vi "tablePartsTracking.vi"(8 "error in (no error)":errorcluster, 10 "Table in":refnum<vi>, 11 "reference in":refnum<class "Project Panels.lvclass">) -> (0 "error out":errorcluster, 3 "reference out":refnum<class "Project Panels.lvclass">)   [LabVIEW 2015, in "Project Panels.lvclass"]
uses:
  Project Panels.lvclass
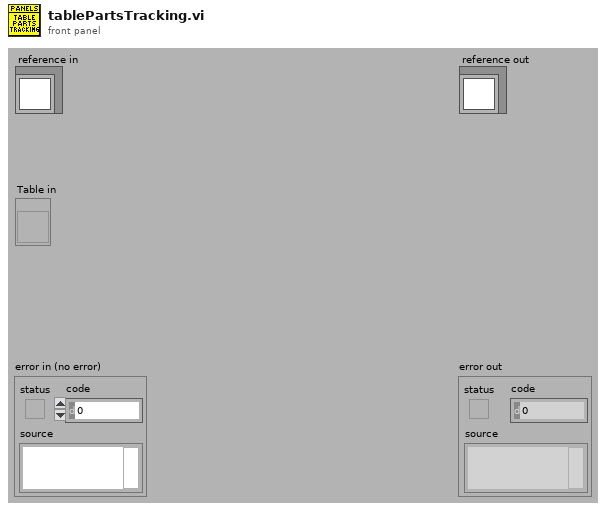
[diagram p1: front panel]
types:
  T1 = enum16{"User-specified Font", "Application Font", "System Font", "Dialog Font"}
  T2 = cluster{"Font Name:":string, "Size":i16, "Strikeout?":bool, "Italic?":bool, "Underline?":bool, "Outline?":bool, "Shadow?":bool, "Bold?":bool}
  T3 = typedef "Project Panels.lvclass/ObjectAttributesRef.ctl" = refnum<data-value>
  T4 = typedef "Project Panels.lvclass/ObjectAttributes.ctl" = cluster{"MyAttribute":dbl, "device_controller_ref":refnum<class "Devices Controller.lvclass">, "file_controller_ref":refnum<class "File Controller.lvclass">, "item_controller_ref":refnum<class "Items Controller.lvclass">, "item_tables":cluster{"checkIN":string[][], "checkOUT":string[][], "storage":string[][]}, "quickbook_table":cluster{"notes":string[][]}, "notification_controller_ref":refnum<class "Notification Controller.lvclass">, "partstracking_controller_ref":refnum<class "PartsTracking Controller.lvclass">, "product_tables":cluster{"k4b2":string[][], "fitmate":string[][], "RMR":string[][], "CPET":string[][], "BP":string[][], "PP":string[][], "k5":string[][], "bb-pft":string[][]}, "rowsColour":u32[], "low_resolution?":bool}
  T5 = cluster{"left":i16, "top":i16, "right":i16, "bottom":i16}
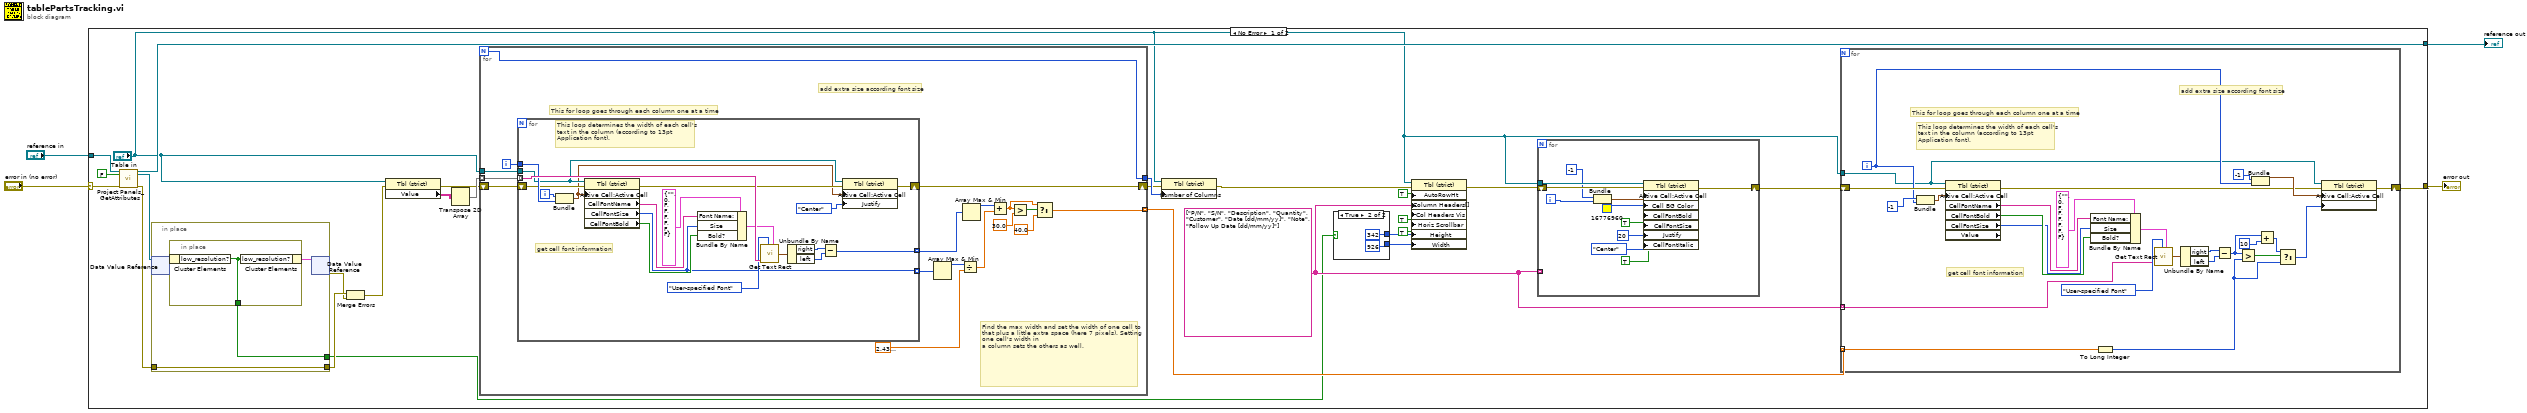
[diagram p0: block diagram]
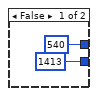
[diagram p2: hidden frame]
diagram:
  n1 = case shown="No Error" "error in (no error)" {
    selector: "error in (no error)" -> [w29 w115]
    tunnel: [w18 w115] -> w3
    tunnel: [w28 w114] -> w1
    tunnel: "reference in" -> [w31 w114]
    frame No Error {
      w14 = string[] ["P/N", "S/N", "Description", "Quantity", "Customer", "Date [dd/mm/yy]", "Note", "Follow Up Date [dd/mm/yy]"] ("Column Header Strings[]")
      n2 = call "Project Panels_GetAttributes.vi"("reference in"=w31, "return data? (T)"=FALSE, "error in (no error)"=w29) -> ("reference out"=w28:refnum<class "Project Panels.lvclass">, "attributes ref"=w6:T3, "error out"=w7:errorcluster)  [unwired: 13 in, 1 out]
      n3 = in-place {
        in-place-border: w7 -> [w33]
        in-place-border: [w33] -> w10
        in-place-border: [w32] -> w5
        n4 = in-place-dvr #1(w6) -> (w34:T4)  [unwired: 1 out]
        n5 = in-place {
          in-place-border: [w36] -> w32
          n6 = in-place-cluster #2(w34) -> ("low_resolution?"=w36:bool)
          n7 = in-place-cluster #2("low_resolution?"=w36) -> (w35:T4)
        }
        n8 = in-place-dvr #1(w35) -> (w9:errorcluster)  [unwired: 1 out]
      }
      n9 = Merge Errors(w10, w9) -> (w8:errorcluster)
      n10 = property on="Property Node" class="Tbl (strict)"(reference="Table in", error in=w8) -> (error out=w23:errorcluster, "Value"=w24:string[][])  [unwired: 1 out]
      n11 = Transpose 2D Array(2D array=w24) -> (transposed array=w25:string[][])
      n12 = for {
        N -> [w86]
        tunnel: w25 -> [w94] mode=indexing
        tunnel: [w86] -> w27
        tunnel: "Table in" -> [w85]
        shift-right: [w79] -> w26
        shift-left: w23 -> [w84]
        tunnel: [w78] -> w11 mode=indexing
        i -> [w92]
        # "add extra size according font size"
        # "Find the max width and set the width of one cell to that plus a little extra space (here 7 pixels). Setting one cell's width in\na column sets the others as well."
        # "This for loop goes through each column one at a time"
        n13 = for {
          tunnel: w94 -> [w113] mode=indexing
          tunnel: [w109] -> w93 mode=indexing
          tunnel: w92 -> [w104]
          tunnel: [w101] -> w90 mode=indexing
          tunnel: w85 -> [w96]
          shift-right: [w98] -> w79
          shift-left: w84 -> [w100]
          i -> [w103]
          # "get cell font information"
          # "This loop determines the width of each cell's\ntext in the column (according to 13pt\nApplication font)."
          n14 = Bundle(w103, w104) -> (w95:cluster{i32, i32})  [unwired: 1 in]
          n15 = property on="Property Node" class="Tbl (strict)"(reference=w96, error in=w100, "Active Cell:Active Cell"=w95) -> (error out=w99:errorcluster, "CellFontName"=w108:string, "CellFontSize"=w101:u32, "CellFontBold"=w107:bool)  [unwired: 1 out]
          n16 = Bundle By Name(cluster=T2 {"Font Name:"="", "Size"=0, "Strikeout?"=FALSE, "Italic?"=FALSE, "Underline?"=FALSE, "Outline?"=FALSE, "Shadow?"=FALSE, "Bold?"=FALSE} ("[user-specified font]"), "Font Name:"=w108, "Size"=w101, "Bold?"=w107) -> (w105:T2)
          n17 = call <vilib>:"Get Text Rect.vi"("desired font(Application)"=T1."User-specified Font", "text"=w113, "[user-specified font]"=w105) -> ("rect"=w112:T5)  [unwired: 6 in]
          n18 = Unbundle By Name(w112) -> ("right"=w111:i16, "left"=w110:i16)
          n19 = Subtract(x=w111, y=w110) -> (x-y=w109:i16)
          n20 = property on="Property Node" class="Tbl (strict)"(reference=w96, error in=w99, "Active Cell:Active Cell"=w95, "Justify"=enum16{"Left", "Center", "Right"}."Center" ("Active Cell:Cell Justification")) -> (error out=w98:errorcluster)  [unwired: 1 out]
        }
        n21 = Array Max & Min(array=w90) -> (max value=w89:u32)  [unwired: 3 out]
        n22 = Divide(x=w89, y=sgl 2.43) -> (x/y=w87:sgl)
        n23 = Array Max & Min(array=w93) -> (max value=w91:i16)  [unwired: 3 out]
        n24 = Add(x=w91, y=w87) -> (x+y=w80:sgl)
        n25 = Greater?(x=w80, y=sgl 30.0) -> (0:w82:bool)
        n26 = Select(t=w80, s=w82, f=sgl 40.0 ("y")) -> (s? t:f=w78:sgl)
      }
      n27 = property on="Property Node" class="Tbl (strict)"(reference="Table in", error in=w26, "Number of Columns"=w27) -> (error out=w19:errorcluster)  [unwired: 1 out]
      n28 = case shown="True" w5 {
        tunnel: [u32 540 ("Size:Height") u32 342 ("Size:Height")] -> w13
        tunnel: [u32 1413 ("Size:Width") u32 926 ("Size:Width")] -> w12
        frame False {
        }
        frame True {
        }
      }
      n29 = property on="Property Node" class="Tbl (strict)"(reference="Table in", error in=w19, "AutoRowHt"=TRUE ("Autosizing Row Height"), "Column Headers[]"=w14, "Col Headers Vis"=TRUE ("Visible Items:Column Headers Visible"), "Horiz Scrollbar"=TRUE ("Visible Items:Horizontal Scrollbar Visible"), "Height"=w13, "Width"=w12) -> (error out=w17:errorcluster)  [unwired: 1 out]
      n30 = for {
        tunnel: "Table in" -> [w49]
        tunnel: w14 -> [_] mode=indexing
        shift-right: [w50] -> w16
        shift-left: w17 -> [w51]
        i -> [w47]
        n31 = Bundle("index"=-1, w47) -> (w48:cluster{"index":i32, i32})  [unwired: 1 in]
        n32 = property on="Property Node" class="Tbl (strict)"(reference=w49, error in=w51, "Active Cell:Active Cell"=w48, "Cell BG Color"=u32 16776960, "CellFontBold"=TRUE ("Active Cell:Cell Font:Bold"), "CellFontSize"=u32 20 ("Active Cell:Cell Font:Size"), "Justify"=enum16{"Left", "Center", "Right"}."Center" ("Active Cell:Cell Justification"), "CellFontItalic"=TRUE ("Active Cell:Cell Font:Italic")) -> (error out=w50:errorcluster)  [unwired: 1 out]
      }
      n33 = for {
        tunnel: "Table in" -> [w57]
        shift-right: [w75] -> w18
        shift-left: w16 -> [w74]
        tunnel: w14 -> [w55] mode=indexing
        tunnel: w11 -> [w53] mode=indexing
        i -> [w63]
        # "get cell font information"
        # "This loop determines the width of each cell's\ntext in the column (according to 13pt\nApplication font)."
        # "add extra size according font size"
        # "This for loop goes through each column one at a time"
        n34 = Bundle("index"=-1, w63) -> (w62:cluster{"index":i32, i32})  [unwired: 1 in]
        n35 = property on="Property Node" class="Tbl (strict)" props=["Active Cell:Active Cell", "CellFontName", "CellFontBold", "CellFontSize", "Value"](reference=w57, error in=w74, "Active Cell:Active Cell"=w62) -> (error out=w54:errorcluster, "CellFontName"=w69:string, "CellFontBold"=w68:bool, "CellFontSize"=w56:u32)  [unwired: 2 out]
        n36 = Bundle By Name(cluster=T2 {"Font Name:"="", "Size"=0, "Strikeout?"=FALSE, "Italic?"=FALSE, "Underline?"=FALSE, "Outline?"=FALSE, "Shadow?"=FALSE, "Bold?"=FALSE} ("[user-specified font]"), "Font Name:"=w69, "Size"=w56, "Bold?"=w68) -> (w66:T2)
        n37 = To Long Integer(number=w53) -> (32bit integer=w52:i32)
        n38 = call <vilib>:"Get Text Rect.vi"("desired font(Application)"=T1."User-specified Font", "text"=w55, "[user-specified font]"=w66) -> ("rect"=w72:T5)  [unwired: 6 in]
        n39 = Unbundle By Name(w72) -> ("right"=w71:i16, "left"=w70:i16)
        n40 = Subtract(x=w71, y=w70) -> (x-y=w60:i16)
        n41 = Greater?(x=w60, y=w52) -> (0:w61:bool)
        n42 = Bundle(-1, w63) -> (w76:cluster{i32, i32})  [unwired: 1 in]
        n43 = Add(x=w60, y=i16 10) -> (x+y=w58:i16)
        n44 = Select(t=w58, s=w61, f=w52) -> (s? t:f=w73:i32)
        n45 = property on="Property Node" class="Tbl (strict)"(reference=w57, error in=w54, "Active Cell:Active Cell"=w76, "Active Cell:Cell Size:Width"=w73) -> (error out=w75:errorcluster)  [unwired: 1 out]
      }
    }
    frame Error {
    }
  }
  "error out" <- w3
  "reference out" <- w1
